vi "FVIR Modbus Setup Part 1.vi"(8 "error in (no error)":errorcluster, 10 "Initialize? in":bool, 11 "Queue in":refnum<queue>) -> (0 "error out":errorcluster, 3 "Queue out":refnum<queue>)   [LabVIEW 2020]
uses:
  Message Queue/Message Cluster.ctl
  Message Queue/Message Queue.lvlib
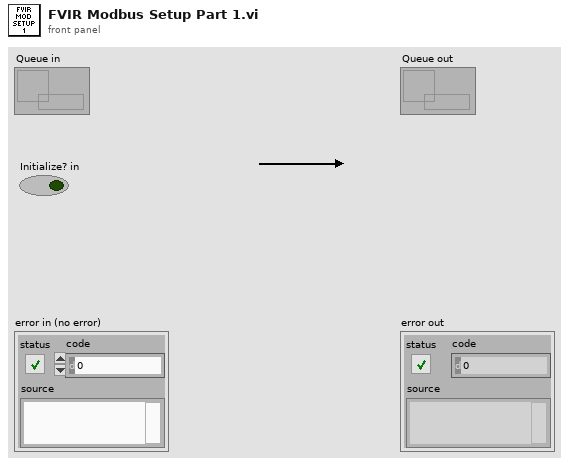
[diagram p1: front panel]
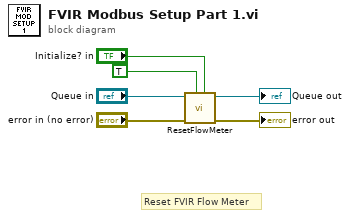
[diagram p0: block diagram]
diagram:
  # "Reset FVIR Flow Meter"
  n1 = call "ResetFlowMeter.vi"("Initialize?"="Initialize? in", "FVIR?"=TRUE, "error in (no error)"="error in (no error)", "Modbus Queue in"="Queue in") -> ("error out"=→"error out":errorcluster, "dup Message Queue"=→"Queue out":refnum<queue>)  [unwired: 6 in]
